vi "voltage_measurement.vi"(8 "error in":errorcluster, 10 "Voltage meas settings":T1={"Physical Channel"="Dev1/ai0", "Min Voltage"=-5.0, "Max Voltage"=5.0, "Terminal Configuration"=-1, "Sample Rate"=1000.0, "Number of Samples"=100} {"Terminal Configuration" items=["default"=-1, "RSE"=10083, "NRSE"=10078, "Differential"=10106, "Pseudodifferential"=12529]}) -> (0 "error out":errorcluster, 2 "Waveform Graph":waveform(dbl)[](graph))   [LabVIEW 2019]
uses:
  <vilib>/DAQmx/configure/timing.llb/DAQmx Timing (Sample Clock).vi
  <vilib>/DAQmx/read.llb/DAQmx Read (Analog 1D Wfm NChan NSamp).vi
  <vilib>/DAQmx/create/channels.llb/DAQmx Create Channel (AI-Voltage-Basic).vi
  ctl_voltage_meas_settings_cluster.ctl
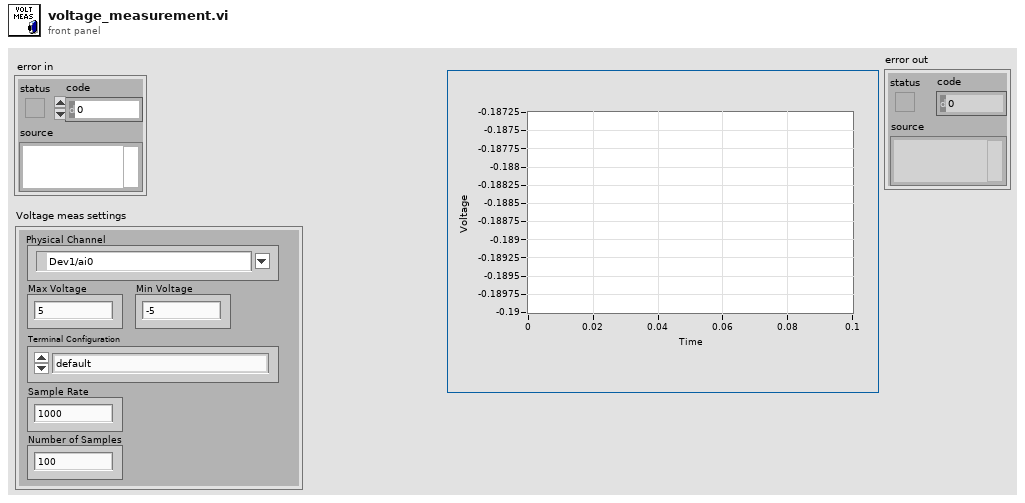
[diagram p1: front panel]
types:
  T1 = typedef "ctl_voltage_meas_settings_cluster.ctl" = cluster{"Physical Channel":tag, "Min Voltage":dbl, "Max Voltage":dbl, "Terminal Configuration":i32, "Sample Rate":dbl, "Number of Samples":i32}
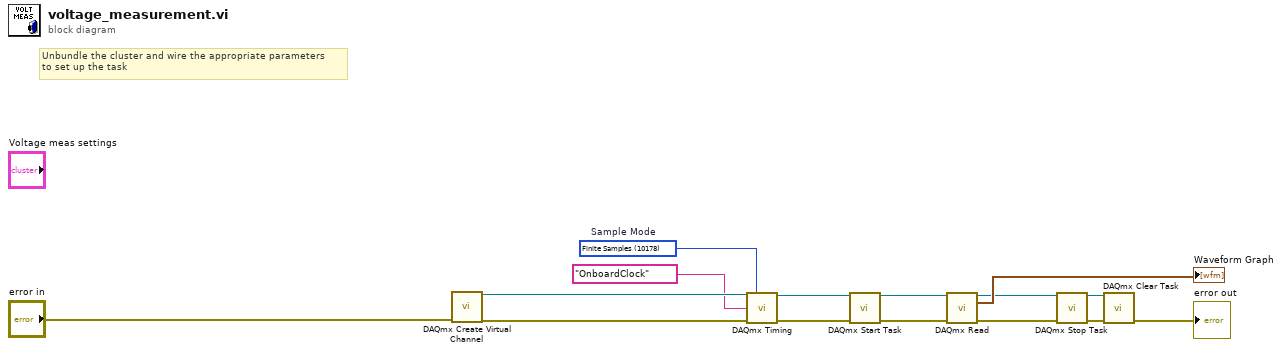
[diagram p0: block diagram]
diagram:
  w15 = 10178 items=["Finite Samples"=10178, "Continuous Samples"=10123, "Hardware Timed Single Point"=12522]  # Sample Mode
  # "Unbundle the cluster and wire the appropriate parameters\nto set up the task"
  n1 = call-poly <vilib>:"DAQmx Create Virtual Channel.vi"("error in"="error in") -> ("task out"=w13:refnum<k21>, "error out"=w14:errorcluster)  [unwired: 13 in]
  n2 = call-poly <vilib>:"DAQmx Timing.vi"("task/channels in"=w13, "sample mode"=w15, "source"=tag "OnboardClock" ("Sample Clock Source"), "error in"=w14) -> ("task out"=w4:refnum<k21>, "error out"=w3:errorcluster)  [unwired: 10 in]
  n3 = call <vilib>:"DAQmx Start Task.vi"("task/channels in"=w4, "error in"=w3) -> ("task out"=w11:refnum<k21>, "error out"=w10:errorcluster)  [unwired: 12 in]
  n4 = call-poly <vilib>:"DAQmx Read.vi"("task/channels in"=w11, "error in"=w10) -> ("task out"=w6:refnum<k21>, "data"=→"Waveform Graph":waveform(dbl)[], "error out"=w5:errorcluster)  [unwired: 11 in]
  n5 = call <vilib>:"DAQmx Stop Task.vi"("task/channels in"=w6, "error in"=w5) -> ("task out"=w8:refnum<k21>, "error out"=w7:errorcluster)  [unwired: 12 in]
  n6 = call <vilib>:"DAQmx Clear Task.vi"("task in"=w8, "error in"=w7) -> ("error out"=→"error out":errorcluster)  [unwired: 13 in]
